vi "全局变量.vi"() -> ()   [LabVIEW 2016, in "多参数状态显示.xctl"]
panel:
  in  "检测值2":dbl[](array[numeric])
  in  "检测值1":dbl[](array[numeric])
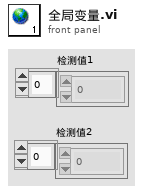
[diagram p1: front panel]
diagram:
